vi "Update Waveform Array Test.vi"() -> ()   [LabVIEW 2015]
panel:
  out "updated wavefrom array":waveform(dbl)[](array[waveform]) caption="更新后波形数组"
  out "min duration":dbl caption="最小时长"
  out "Waveform Array":waveform(dbl)[](array[waveform]) caption="波形数据"
  out "error out":errorcluster caption="错误输出"
  in  "Timestamp":timestamp caption="时间标识"
  in  "sampling period (s)":dbl caption="采样周期 (s)"
  in  "samples to write":dbl[](array[numeric]) caption="待写入采样点"
  in  "error in (no error)":errorcluster caption="错误输入（无错误）"
  in  "channel info array":cluster{"Module":string, "Channel":string}[](array[cluster]) caption="通道信息数组"
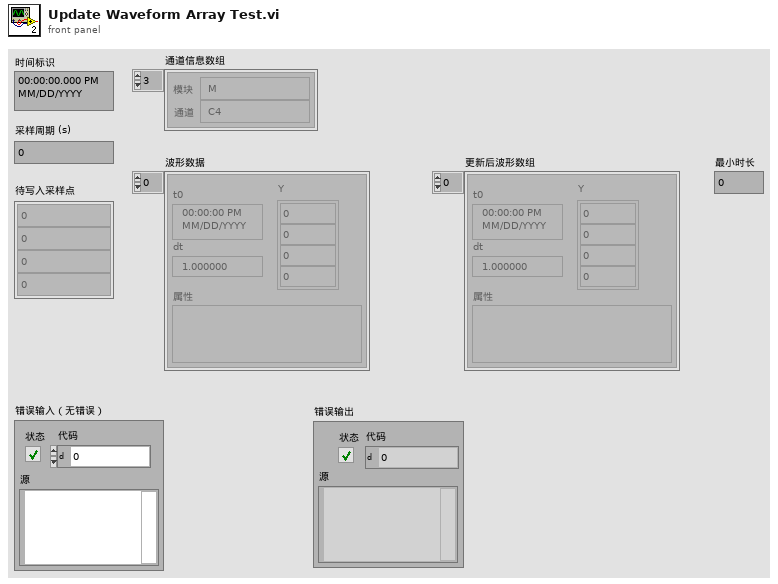
[diagram p1: front panel]
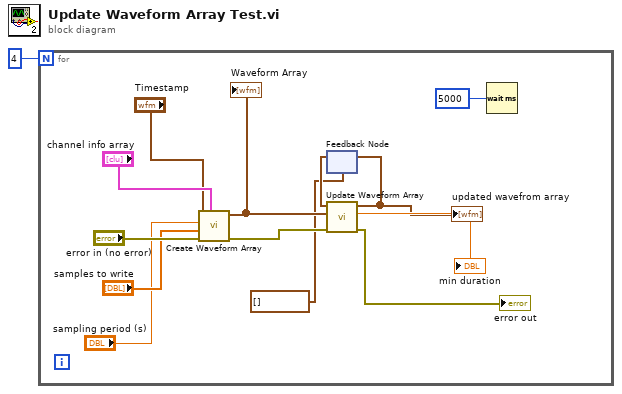
[diagram p0: block diagram]
diagram:
  n1 = for {
    N: 4 -> [_]
    n2 = call "Create Waveform Array.vi"("channel info array"="channel info array", "error in (no error)"="error in (no error)", "samples to write"="samples to write", "sampling period (s)"="sampling period (s)", "Timestamp"="Timestamp") -> ("error out"=w9:errorcluster, "Waveform Array"=w7:waveform(dbl)[])  [unwired: 5 in]
    "Waveform Array" <- w7
    n3 = feedback #1(waveform(dbl)[] []) -> (w4:waveform(dbl)[])
    n4 = call "Update Waveform Array.vi"("error in (no error)"=w9, "new waveform array"=w7, "original waveform array"=w4) -> ("error out"=→"error out":errorcluster, "min duration"=→"min duration":dbl, "updated wavefrom array"=w5:waveform(dbl)[])  [unwired: 6 in]
    "updated wavefrom array" <- w5
    n5 = feedback-in #1(w5) -> ()
    n6 = Wait (ms)(milliseconds to wait=u32 5000 ("等待时间（毫秒）")) -> ()  [unwired: 1 out]
  }
